vi "ZCAN_ParsesFrame.vi"(5 "ZCAN_Receive_Data":T1, 11 "error in (no error)":errorcluster caption="错误输入（无错误）") -> (3 "帧格式":string, 4 "帧类型":string, 6 "ID":u32, 8 "data_len":u8, 10 "data":u8[](array[numeric]), 15 "error out":errorcluster caption="错误输出")   [LabVIEW 2018]
doc: "解析单帧CAN报文。"
panel:
  in  "空数组":u8[](array[numeric])
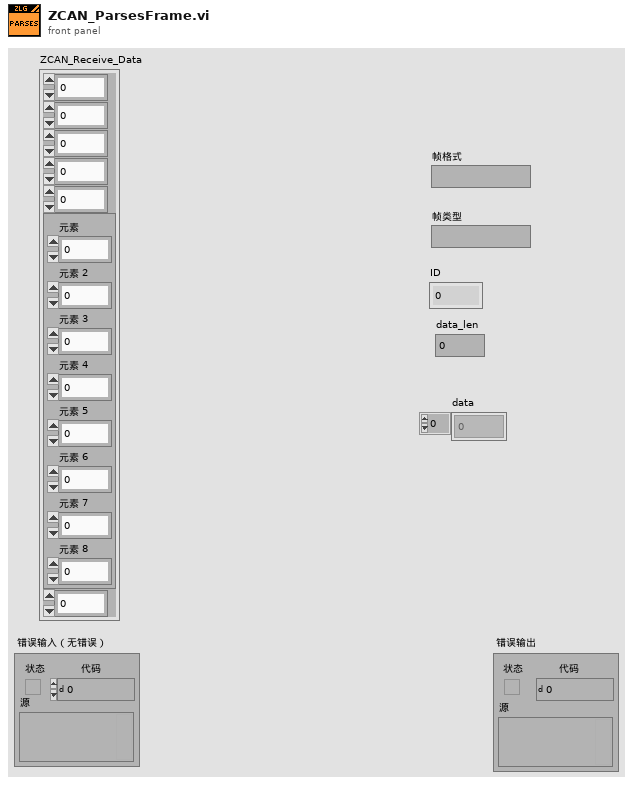
[diagram p1: front panel]
types:
  T1 = cluster{u32, u8, u8, u8, u8, cluster{"元素":u8, "元素 2":u8, "元素 3":u8, "元素 4":u8, "元素 5":u8, "元素 6":u8, "元素 7":u8, "元素 8":u8}, u64}
  T2 = cluster{"元素":u8, "元素 2":u8, "元素 3":u8, "元素 4":u8, "元素 5":u8, "元素 6":u8, "元素 7":u8, "元素 8":u8}
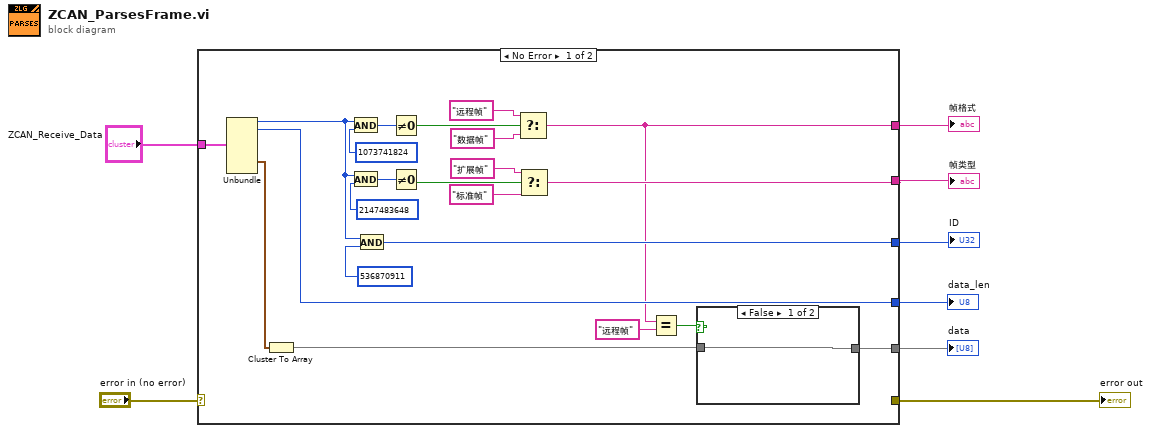
[diagram p0: block diagram]
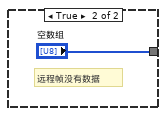
[diagram p2: hidden frame]
diagram:
  n1 = case shown="No Error" "error in (no error)" {
    selector: "error in (no error)" -> [_ w33]
    tunnel: [_ w33] -> w7
    tunnel: "ZCAN_Receive_Data" -> [w25 _]
    tunnel: [w23 _] -> w1
    tunnel: [w12 _] -> w3
    tunnel: [w14 _] -> w2
    tunnel: [w15 _] -> w5
    tunnel: [w10 _] -> w4
    frame No Error {
      n2 = Unbundle(w25) -> (w24:u32, w15:u8, w22:T2)  [unwired: 4 out]
      n3 = Cluster To Array(cluster=w22) -> (array=w9:u8[])
      n4 = And(x=w24, y=u32 1073741824) -> (x .and. y?=w26:u32)
      n5 = And(x=w24, y=u32 2147483648) -> (x .and. y?=w27:u32)
      n6 = And(x=w24, y=u32 536870911) -> (x .and. y?=w23:u32)
      n7 = Not Equal To 0?(x=w26) -> (x != 0?=w17:bool)
      n8 = Not Equal To 0?(x=w27) -> (x != 0?=w16:bool)
      n9 = Select(t="远程帧", s=w17, f="数据帧") -> (s? t:f=w12:string)
      n10 = Select(t="扩展帧", s=w16, f="标准帧") -> (s? t:f=w14:string)
      n11 = Equal?(x=w12, y="远程帧") -> (x = y?=w11:bool)
      n12 = case shown="False" w11 {
        tunnel: [w31 "空数组"] -> w10
        tunnel: w9 -> [w31 _]
        frame False {
        }
        frame True {
          # "远程帧没有数据"
        }
      }
    }
    frame Error {
    }
  }
  "error out" <- w7
  "ID" <- w1
  "帧格式" <- w3
  "帧类型" <- w2
  "data_len" <- w5
  "data" <- w4
